vi "AIs-Freq.vi"(6 "Slot":T1, 8 "error in":errorcluster, 10 "Mode":string, 11 "CHs":string[](array[string])) -> (0 "error out":errorcluster, 2 "RMS value":dbl caption="均方根值" format="%0.2p", 3 "波形图":waveform(dbl)[](graph))   [LabVIEW 2013]
uses:
  SystemCode/SysControl/Slot.ctl
  <vilib>/DAQmx/read.llb/DAQmx Read (Analog 1D Wfm NChan NSamp).vi
  SourceCode/GlobalValue.vi
  <vilib>/DAQmx/create/channels.llb/DAQmx Create Channel (AI-Voltage-Basic).vi
  <vilib>/DAQmx/configure/timing.llb/DAQmx Timing (Sample Clock).vi
  <vilib>/addons/Sound and Vibration/svt_Distortion/SVT THD+N (Time) (1 Ch).vi
  <vilib>/measure/matone.llb/SINAD Analyzer 1 Chan.vi
  <vilib>/measure/madcrms.llb/Basic Averaged DC-RMS for 1 Chan.vi
  <vilib>/DAQmx/miscellaneous.llb/DAQmx Fill In Error Info.vi
  <vilib>/measure/NI_MAPro.lvlib
  <vilib>/addons/Sound and Vibration/svt_Distortion/SoundVib_Distortion.lvlib
panel:
  out "THD+N 2":dbl format="%.2f"
  out "THD Plus Noise":dbl caption="总谐波失真叠加噪声" format="%.2p"
  out "SINAD (dB)":dbl format="%.2p"
  out "THD+N":dbl format="%.2f"
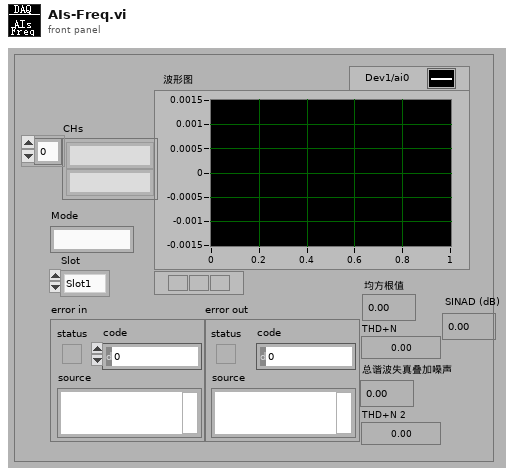
[diagram p1: front panel]
types:
  T1 = typedef "Slot.ctl" = enum16{"Slot1", "Slot2", "Slot3", "Slot4"}
  T2 = cluster{"THD+N units":enum16{"dB", "linear ratio", "%"}, "detected fundamental amplitude units":enum16{"EU rms", "EU peak", "EU peak-peak"}}
  T3 = typedef "DAQConfig.ctl" = cluster{"DIO":string[][], "AO":string[][], "AI":string[][]}
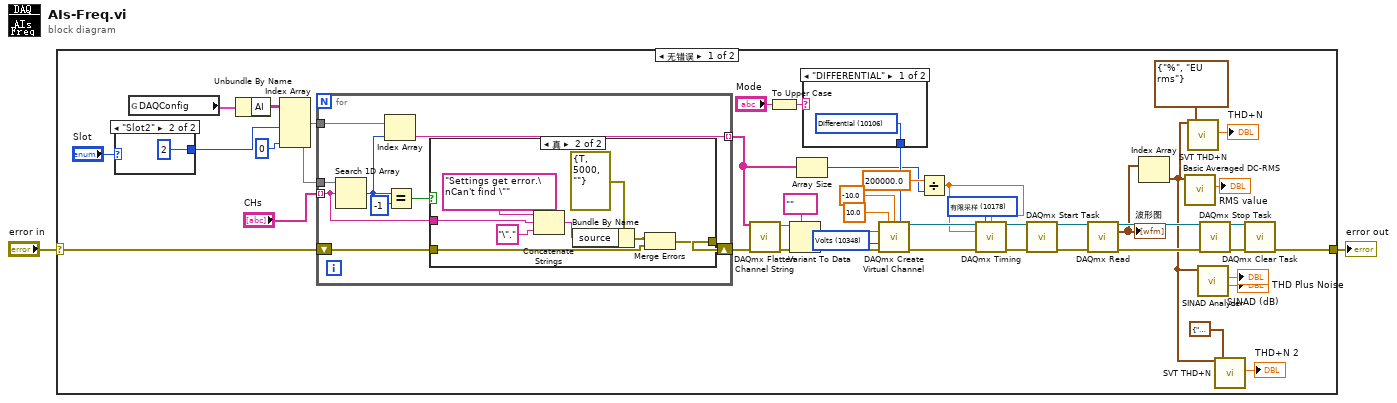
[diagram p0: block diagram]
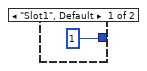
[diagram p2: hidden frame]
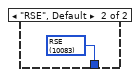
[diagram p4: hidden frame]
diagram:
  n1 = case shown="无错误" "error in" {
    selector: "error in" -> [w32 w71]
    tunnel: [w48 w71] -> w2
    frame No Error {
      w28 = 10178 items=["有限采样"=10178, "连续采样"=10123, "硬件定时单点"=12522] ("sample mode")
      w43 = 10348 items=["Volts"=10348, "From Custom Scale"=10065] ("units")
      n2 = case shown="\"Slot2\"" "Slot" {
        tunnel: [1 ("索引 (行)") 2 ("索引 (行)")] -> w14
        frame "Slot1", Default {
        }
        frame "Slot2" {
        }
      }
      n3 = global read "GlobalValue.vi" "DAQConfig"() -> (w12:T3)
      n4 = Unbundle By Name(w12) -> ("AI"=w39:string[][])
      n5 = Index Array(array=w39, index (col) #1=w14, index (col) #2=0 ("索引 (列)")) -> (element #1=w37:string[], element #2=w36:string[])  [unwired: 2 in]
      n6 = for {
        tunnel: w37 -> [w57]
        tunnel: w36 -> [w56]
        tunnel: "CHs" -> [w54] mode=indexing
        tunnel: [w51] -> w18 mode=indexing
        shift-right: [w53] -> w20
        shift-left: w32 -> [w52]
        n7 = Search 1D Array(1D array=w56, element=w54) -> (index of element=w59:i32)  [unwired: 1 in]
        n8 = Index Array(array=w57, index=w59) -> (element=w51:string)
        n9 = Equal?(x=w59, y=-1) -> (x = y?=w55:bool)
        n10 = case shown="真" w55 {
          tunnel: w52 -> [w60 w64]
          tunnel: [w60 w63] -> w53
          tunnel: w54 -> [_ w62]
          frame False {
          }
          frame True {
            n11 = Concatenate Strings("Settings get error.\nCan't find \"" ("message"), w62, "\"." ("string")) -> (w67:string)
            n12 = Bundle By Name(cluster=errorcluster {"status"=TRUE, "code"=5000, "source"=""} ("error in 1 (no error)"), "source"=w67) -> (w66:errorcluster)
            n13 = Merge Errors(w66, w64) -> (w63:errorcluster)
          }
        }
      }
      n14 = call <vilib>:"DAQmx Flatten Channel String.vi"("names in"=w18, "error in"=w20) -> ("names out"=w19:string, "error out"=w21:errorcluster)  [unwired: 12 in]
      n15 = To Upper Case(1:"Mode") -> (0:w30:string)
      n16 = Variant To Data(error in=w21, type=tag "" ("lines"), Variant=w19) -> (data=w34:tag, error out=w33:errorcluster)
      n17 = Array Size(array=w18) -> (size(s)=w16:i32)
      n18 = case shown="\"DIFFERENTIAL\"" w30 {
        tunnel: [w69 w70] -> w29
        frame "DIFFERENTIAL" {
          w69 = 10106 items=["default"=-1, "RSE"=10083, "NRSE"=10078, "Differential"=10106, "Pseudodifferential"=12529] ("input terminal configuration")
        }
        frame "RSE", Default {
          w70 = 10083 items=["default"=-1, "RSE"=10083, "NRSE"=10078, "Differential"=10106, "Pseudodifferential"=12529] ("input terminal configuration")
        }
      }
      n19 = call-poly <vilib>:"DAQmx Create Virtual Channel.vi"("maximum value"=10.0, "minimum value"=-10.0, "input terminal configuration"=w29, "physical channels"=w34, "units"=w43, "error in"=w33) -> ("task out"=w27:refnum<k21>, "error out"=w25:errorcluster)  [unwired: 8 in]
      n20 = Divide(x=200000.0, y=w16) -> (x/y=w13:dbl)
      n21 = call-poly <vilib>:"DAQmx Timing.vi"("task/channels in"=w27, "sample mode"=w28, "samples per channel"=w13, "rate"=w13, "error in"=w25) -> ("task out"=w26:refnum<k21>, "error out"=w24:errorcluster)  [unwired: 2 in, 7 out]
      n22 = call <vilib>:"DAQmx Start Task.vi"("task/channels in"=w26, "error in"=w24) -> ("task out"=w47:refnum<k21>, "error out"=w46:errorcluster)  [unwired: 12 in]
      n23 = call-poly <vilib>:"DAQmx Read.vi"("task/channels in"=w47, "error in"=w46) -> ("task out"=w42:refnum<k21>, "data"=w11:waveform(dbl)[], "error out"=w23:errorcluster)  [unwired: 11 in]
      "波形图" <- w11
      n24 = Index Array(array=w11) -> (element=w5:waveform(dbl))  [unwired: 1 in]
      n25 = call-poly <vilib>:"Basic Averaged DC-RMS.vi"("signal in"=w5) -> ("RMS value"=→"RMS value":dbl)  [unwired: 7 in, 3 out]
      n26 = call-poly <vilib>:"SVT THD+N.vi"("scaled signal [EU]"=w5, "desired units"=T2 {"THD+N units"=enum."%", "detected fundamental amplitude units"=enum."EU rms"}) -> ("THD+N"=→"THD+N":dbl)  [unwired: 12 in, 5 out]
      n27 = call-poly <vilib>:"SINAD Analyzer.vi"("signal in"=w5) -> ("THD Plus Noise"=→"THD Plus Noise":dbl, "SINAD (dB)"=→"SINAD (dB)":dbl)  [unwired: 5 in, 4 out]
      n28 = call <vilib>:"DAQmx Stop Task.vi"("task/channels in"=w42, "error in"=w23) -> ("task out"=w45:refnum<k21>, "error out"=w44:errorcluster)  [unwired: 12 in]
      n29 = call-poly <vilib>:"SVT THD+N.vi"("scaled signal [EU]"=w5, "desired units"=T2 {"THD+N units"=enum."%", "detected fundamental amplitude units"=enum."EU rms"}) -> ("THD+N"=→"THD+N 2":dbl)  [unwired: 12 in, 5 out]
      n30 = call <vilib>:"DAQmx Clear Task.vi"("task in"=w45, "error in"=w44) -> ("error out"=w48:errorcluster)  [unwired: 13 in]
    }
    frame Error {
    }
  }
  "error out" <- w2
